vi "Ketihley_6221_read_data.vi"(0 "refnum":refnum<file>) -> ()   [LabVIEW 2016]
uses:
  Global/Global Variables/Data_Display_global.vi
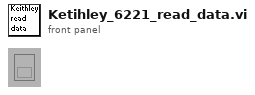
[diagram p1: front panel]
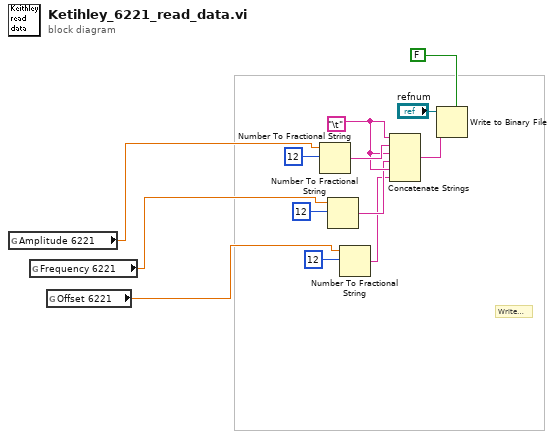
[diagram p0: block diagram]
diagram:
  w3 = "\t"
  # "Write File"
  n1 = global read "Data_Display_global.vi" "Amplitude 6221"() -> (w8:dbl)
  n2 = global read "Data_Display_global.vi" "Frequency 6221"() -> (w5:dbl)
  n3 = global read "Data_Display_global.vi" "Offset 6221"() -> (w4:dbl)
  n4 = Number To Fractional String(number=w8, precision (6)=i16 12) -> (F-format string=w11:string)  [unwired: 2 in]
  n5 = Number To Fractional String(number=w5, precision (6)=i16 12) -> (F-format string=w2:string)  [unwired: 2 in]
  n6 = Number To Fractional String(number=w4, precision (6)=i16 12) -> (F-format string=w1:string)  [unwired: 2 in]
  n7 = Concatenate Strings(w3, w11, w3, w2, w3, w1) -> (w12:string)
  n8 = Write to Binary File ("Write File")(file (use dialog)="refnum", data=w12, 5:FALSE ("prepend array or string size? (T)")) -> ()  [unwired: 3 in, 3 out]
